vi "downsample 1D array - I16 to F32.vi"(2 "Ave N":dbl, 3 "Array In":i16[](array[numeric])) -> (1 "Array Out":sgl[](array[numeric]))   [LabVIEW 2014]
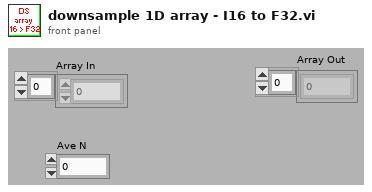
[diagram p1: front panel]
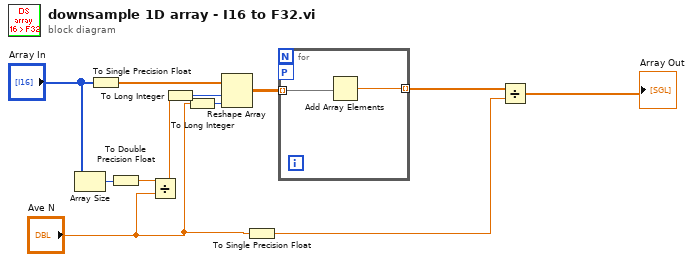
[diagram p0: block diagram]
diagram:
  n1 = Array Size(array="Array In") -> (size(s)=w11:i32)
  n2 = To Single Precision Float(number="Array In") -> (single precision float=w8:sgl[])
  n3 = To Double Precision Float(number=w11) -> (double precision float=w7:dbl)
  n4 = Divide(x=w7, y="Ave N") -> (x/y=w10:dbl)
  n5 = To Long Integer(number=w10) -> (32bit integer=w6:i32)
  n6 = To Long Integer(number="Ave N") -> (32bit integer=w5:i32)
  n7 = Reshape Array(w8, w6, w5) -> (w9:sgl[][])
  n8 = To Single Precision Float(number="Ave N") -> (single precision float=w1:sgl)
  n9 = for {
    tunnel: w9 -> [w14] mode=indexing
    tunnel: [w13] -> w4 mode=indexing
    workers-P: _ -> [_]
    n10 = Add Array Elements(numeric array=w14) -> (sum=w13:sgl)
  }
  n11 = Divide(x=w4, y=w1) -> (x/y=→"Array Out":sgl[])
